vi "DHE_GoExpose.vi"(2 "error in":errorcluster, 4 "fd":i32) -> (0 "error out":errorcluster)   [LabVIEW 2016]
uses:
  DBSHAND/private/vis/DatabaseHand_Element_Set(I32).vi
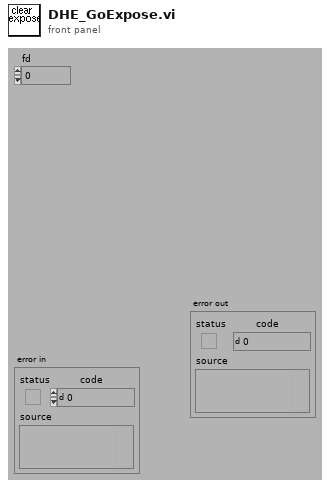
[diagram p1: front panel]
types:
  T1 = typedef "DatabaseHand_RefNum.ctl" = refnum<vi>
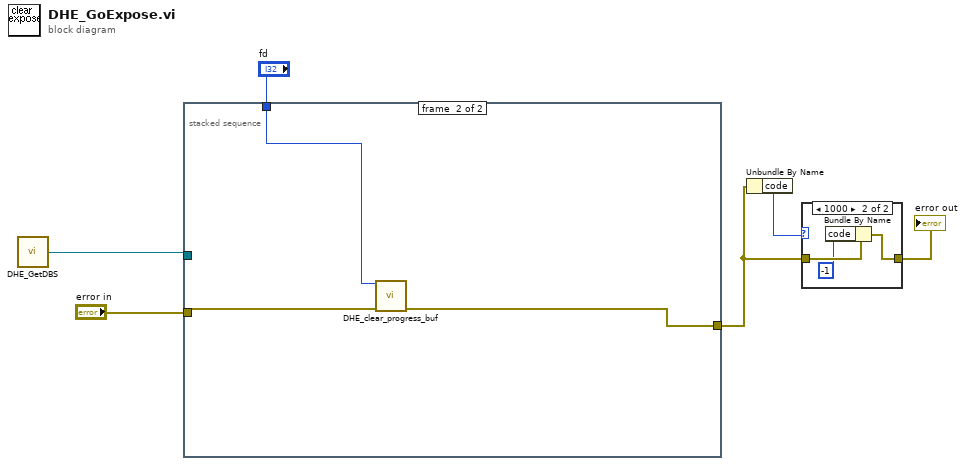
[diagram p0: block diagram]
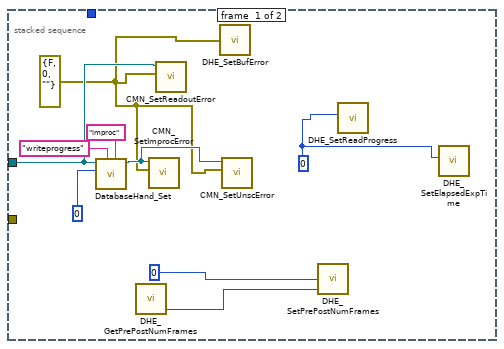
[diagram p3: hidden frame]
diagram:
  n1 = call "DHE_GetDBS.vi"() -> ("DHE_DBSRef"=w1:T1)  [unwired: 9 out]
  n2 = stacked-sequence {
    tunnel: "fd" -> [_ w18]
    tunnel: "error in" -> [_ w17]
    tunnel: [_ w16] -> w3
    tunnel: w1 -> [w12 _]
    frame #0 {
      w9 = errorcluster {"status"=FALSE, "code"=0, "source"=""} ("readout Error")
      w8 = 0
      n3 = call-poly "DatabaseHand_Set.vi"("group"="improc", "name"="writeprogress" ("value"), "value"=0, "Database RefNum in"=w12) -> ("Database RefNum out"=w11:T1)  [unwired: 4 in, 3 out]
      n4 = call "DHE_GetPrePostNumFrames.vi"() -> ("DHE_PostExpose"=w7:i32)  [unwired: 9 out]
      n5 = call "CMN_SetImprocError.vi"("improc error"=w9, "Database RefNum in"=w11) -> ()  [unwired: 1 in, 9 out]
      n6 = call "CMN_SetReadoutError.vi"("readout error"=w9, "Database RefNum in"=w12) -> ()  [unwired: 1 in, 9 out]
      n7 = call "DHE_SetBufError.vi"("DHE_BufError"=w9) -> ()  [unwired: 9 out]
      n8 = call "CMN_SetUnscError.vi"("unsc error"=w9, "Database RefNum in"=w11) -> ()  [unwired: 1 in, 9 out]
      n9 = call "DHE_SetPrePostNumFrames.vi"("DHE_PreExpose"=u16 0 ("pre expose frames"), "DHE_PostExpose"=w7) -> ()  [unwired: 8 out]
      n10 = call "DHE_SetReadProgress.vi"("ReadProgress"=w8) -> ()  [unwired: 11 out]
      n11 = call "DHE_SetElapsedExpTime.vi"("ElapsedExpTime"=w8) -> ()  [unwired: 11 out]
    }
    frame #1 {
      n12 = call "DHE_clear_progress_buf.vi"("fd"=w18, "error in (no error)"=w17) -> ("error out"=w16:errorcluster)  [unwired: 13 out]
    }
  }
  n13 = Unbundle By Name(w3) -> ("code"=w4:i32)
  n14 = case shown="1000" w4 {
    tunnel: w3 -> [w19 w22]
    tunnel: [w19 w21] -> w2
    frame Default {
    }
    frame 1000 {
      n15 = Bundle By Name(cluster=w22, "code"=-1) -> (w21:errorcluster)
    }
  }
  "error out" <- w2
